vi "InSSM.vi"(7 "Set":bool, 11 "InSSM":bool) -> (3 "SSM State":bool)   [LabVIEW 2018, in "Test.lvclass"]
doc: "Functional global variable that records if the SSM is currently in operation or has exited."
uses:
  Test.lvclass
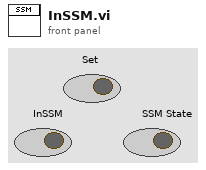
[diagram p1: front panel]
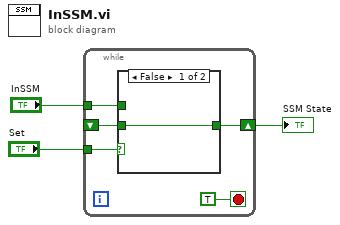
[diagram p0: block diagram]
diagram:
  n1 = while {
    shift-right: [w5] -> w1
    shift-left: _ -> [w4]
    tunnel: "Set" -> [w7]
    tunnel: "InSSM" -> [w6]
    stop <- TRUE stop-if-true
    n2 = case shown="False" w7 {
      tunnel: w6 -> [_ w10]
      tunnel: [w9 w10] -> w5
      tunnel: w4 -> [w9 _]
      frame False {
      }
      frame True {
      }
    }
  }
  "SSM State" <- w1
